vi "Mark Element Changed.vi"(8 "error in (no error)":errorcluster, 10 "Index":i32, 11 "Config Manager in":refnum<class "Config Manager.lvclass">) -> (0 "error out":errorcluster, 3 "Config Manager out":refnum<class "Config Manager.lvclass">)   [LabVIEW 2020, in "CDM-Config.lvlib" / "Config Manager.lvclass"]
uses:
  Config Manager.lvclass
  Config Manager.lvclass/Config Manager.ctl
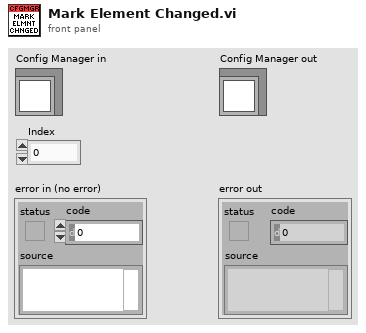
[diagram p1: front panel]
types:
  T1 = typedef "CDM-Config.lvlib/Config Manager.lvclass/Ref Data.ctl" = cluster{"Elements":refnum<class "Config Element.lvclass">[], "Name Separator":string, "Hierarchy Map":map{string[], i32}, "Meta Name Map":map{string, i32[]}, "Element Map":map{refnum<class "Config Element.lvclass">, i32}, "Changed":bool[]}
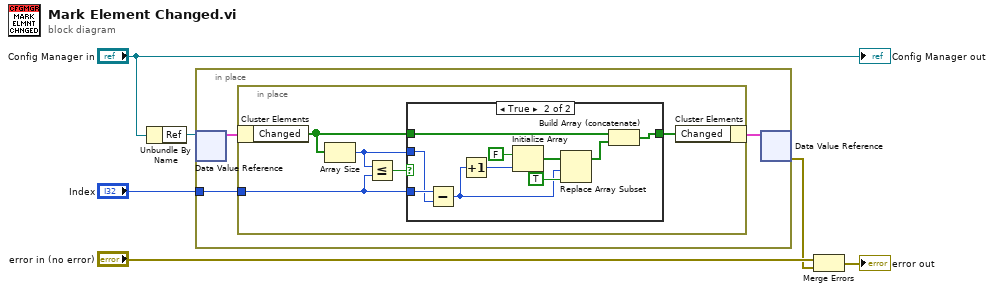
[diagram p0: block diagram]
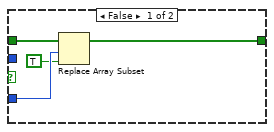
[diagram p2: hidden frame]
diagram:
  n1 = Unbundle By Name("Config Manager in") -> ("Ref"=w5:refnum<data-value>)
  n2 = in-place {
    in-place-border: "Index" -> [w7]
    n3 = in-place-dvr #1(w5) -> (w9:T1)  [unwired: 1 out]
    n4 = in-place {
      in-place-border: w7 -> [w11]
      n5 = in-place-cluster #2(w9) -> ("Changed"=w14:bool[])
      n6 = Array Size(array=w14) -> (size(s)=w12:i32)
      n7 = Less Or Equal?(x=w12, y=w11) -> (x <= y?=w13:bool)
      n8 = case shown="True" w13 {
        tunnel: w14 -> [w18 w21]
        tunnel: w12 -> [_ w27]
        tunnel: w11 -> [w17 w28]
        tunnel: [w15 w19] -> w10
        frame False {
          n9 = Replace Array Subset(array=w18, new element=TRUE ("new element/subarray"), index=w17) -> (w15:bool[])
        }
        frame True {
          n10 = Subtract(x=w28, y=w27) -> (x-y=w22:i32)
          n11 = Increment(x=w22) -> (x+1=w26:i32)
          n12 = Initialize Array(FALSE, w26) -> (w24:bool[])
          n13 = Replace Array Subset(array=w24, new element=TRUE ("new element/subarray"), index=w22) -> (w20:bool[])
          n14 = Build Array (concatenate)(w21, w20) -> (w19:bool[])
        }
      }
      n15 = in-place-cluster #2("Changed"=w10) -> (w8:T1)
    }
    n16 = in-place-dvr #1(w8) -> (w1:errorcluster)  [unwired: 1 out]
  }
  n17 = Merge Errors("error in (no error)", w1) -> (→"error out":errorcluster)
  "Config Manager out" <- "Config Manager in"
